vi "CTRE_Phoenix_CANcoder_GetLastTimestamp.vi"(8 "error in":errorcluster, 11 "CTRE_CANcoder_DeviceRef":T1) -> (0 "error out":errorcluster, 2 "Last Timestamp":dbl, 3 "CTRE_CANcoder_DeviceRef":T1)   [LabVIEW 2020]
doc: "Get the timestamp of the CAN frame retrieved in the last called get routine."
uses:
  <vilib>/Rock Robotics/WPI/ThirdParty/Phoenix-LabVIEW/CANCoder/Controls/CTRE_Phoenix_CANcoder_DeviceRef.ctl
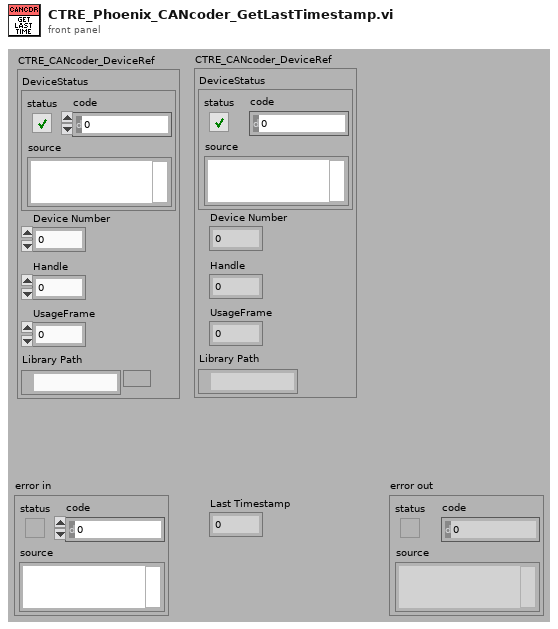
[diagram p1: front panel]
types:
  T1 = typedef "CTRE_Phoenix_CANcoder_DeviceRef.ctl" = cluster{"DeviceStatus":errorcluster, "Device Number":u8, "Handle":u64, "UsageFrame":u32, "Library Path":path}
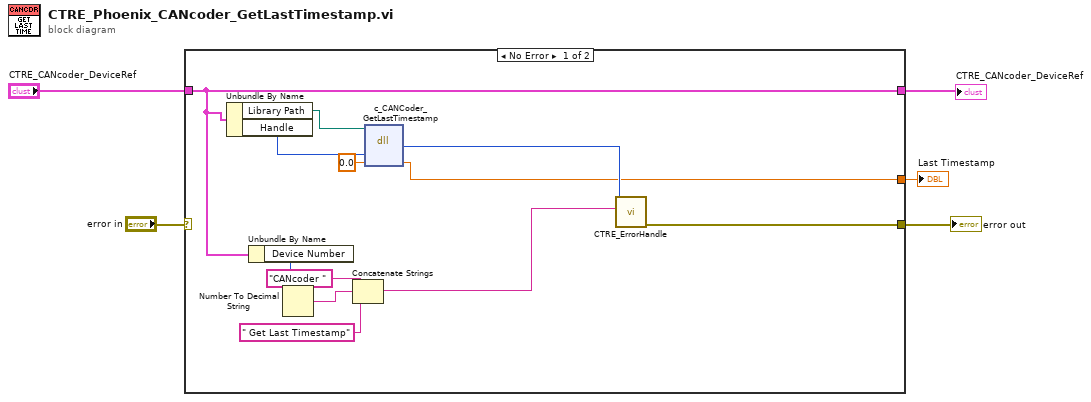
[diagram p0: block diagram]
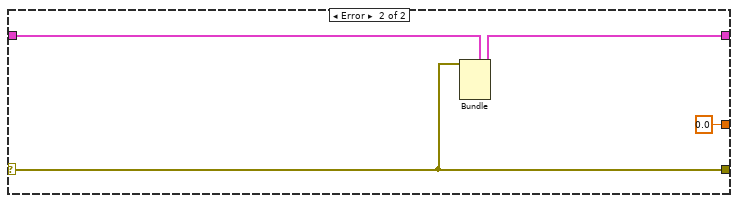
[diagram p2: hidden frame]
diagram:
  n1 = case shown="No Error" "error in" {
    selector: "error in" -> [_ w20]
    tunnel: "CTRE_CANcoder_DeviceRef" -> [w10 w21]
    tunnel: [w17 w20] -> w5
    tunnel: [w10 w19] -> w2
    tunnel: [w6 0.0 ("timestamp")] -> w1
    frame No Error {
      n2 = Unbundle By Name(w10) -> ("Library Path"=w9:path, "Handle"=w8:u64)
      n3 = Unbundle By Name(w10) -> ("Device Number"=w13:u8)
      n4 = Number To Decimal String(number=w13) -> (decimal integer string=w15:string)  [unwired: 1 in]
      n5 = Concatenate Strings("CANcoder " ("string"), w15, " Get Last Timestamp" ("string")) -> (w11:string)
      n6 = dll-call lib="?" fn="c_CANCoder_GetLastTimestamp"(path in=w9, "handle"=w8, "timestamp"=0.0) -> ("return type"=w12:i32, "timestamp"=w6:dbl)  [unwired: 3 in, 2 out]
      n7 = call <vilib>:"CTRE_ErrorHandle.vi"("origin"=w11, "code"=w12) -> ("error out"=w17:errorcluster)  [unwired: 9 in]
    }
    frame Error {
      n8 = Bundle(cluster=w21, "DeviceStatus"=w20) -> (w19:T1)  [unwired: 4 in]
    }
  }
  "error out" <- w5
  "Last Timestamp" <- w1
  "CTRE_CANcoder_DeviceRef" <- w2
